vi "Receive.vi"(8 "error in (no error)":errorcluster, 9 "timeout in ms (-1)":i32=-1, 11 "QueueMessenger in":refnum<class "QueueMessenger.lvclass">) -> (0 "error out":errorcluster, 1 "timed out?":bool, 2 "Message":refnum<class "MSG.lvclass">, 3 "QueueMessenger out":refnum<class "QueueMessenger.lvclass">)   [LabVIEW 2011, in "Messenging.lvlib" / "QueueMessenger.lvclass"]
uses:
  QueueMessenger.lvclass
  TextVarientMessage/MSG.lvclass
  QueueMessenger.lvclass/QueueMessenger.ctl
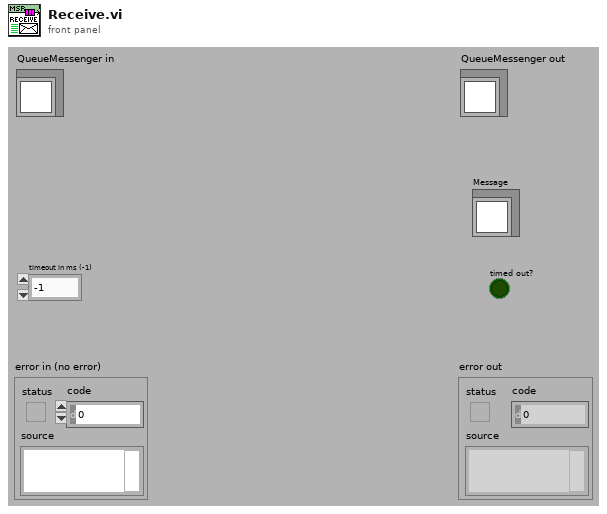
[diagram p1: front panel]
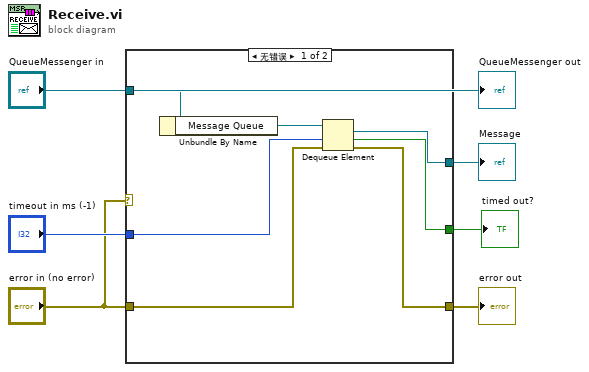
[diagram p0: block diagram]
diagram:
  n1 = case shown="无错误" "error in (no error)" {
    tunnel: "QueueMessenger in" -> [w13 _]
    tunnel: "timeout in ms (-1)" -> [w11 _]
    tunnel: [w10 _] -> w4
    tunnel: [w9 _] -> w3
    tunnel: "error in (no error)" -> [w8 w14]
    tunnel: [w7 w14] -> w2
    frame No Error {
      n2 = Unbundle By Name(w13) -> ("Message Queue"=w12:refnum<queue>)
      n3 = Dequeue Element(queue=w12, timeout in ms (-1)=w11, error in (no error)=w8) -> (element=w10:refnum<class "MSG.lvclass">, timed out?=w9:bool, error out=w7:errorcluster)  [unwired: 1 out]
    }
    frame Error {
    }
  }
  "error out" <- w2
  "Message" <- w4
  "timed out?" <- w3
  "QueueMessenger out" <- "QueueMessenger in"
